vi "Skip Header.vi"(6 "transpose (yes:T)":bool=TRUE, 8 "delimiter (Tab)":string="\t", 9 "number of rows (all:-1)":i32=-1, 10 "number of header lines":i32, 11 "Input File Name":path) -> (0 "Header":string, 1 "header length":i32, 3 "all rows":dbl[][](array[numeric]) format="%_5e", 5 "new file path (Not A Path if cancelled)":path)   [LabVIEW 2018]
uses:
  <vilib>/Utility/file.llb/Read From Spreadsheet File (DBL).vi
panel:
  in  "Numeric":dbl
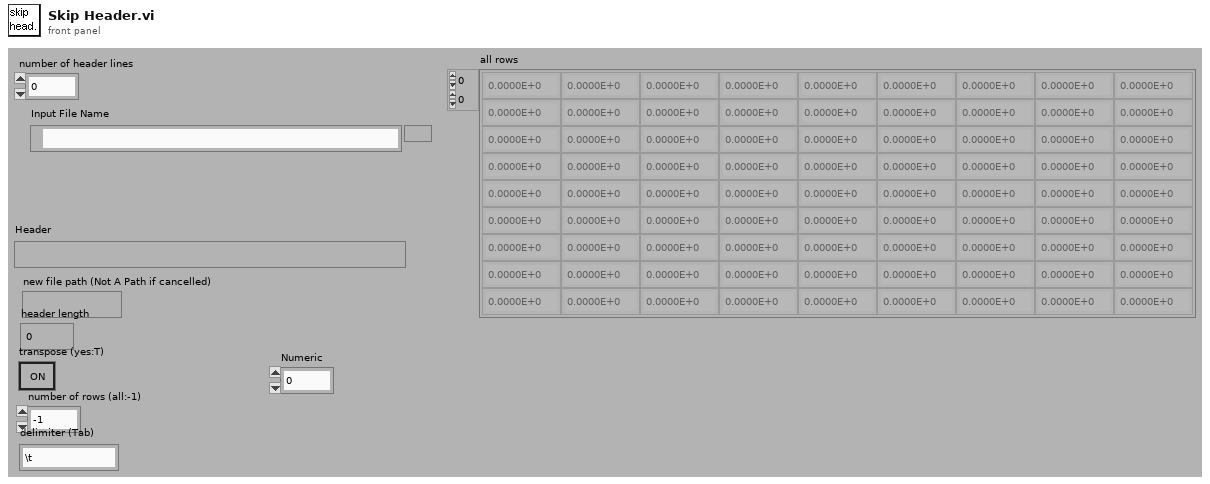
[diagram p1: front panel]
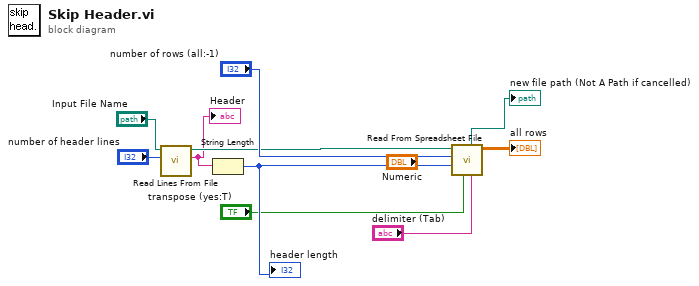
[diagram p0: block diagram]
diagram:
  n1 = call <vilib>:"Read Lines From File.vi"("file path (dialog if empty)"="Input File Name", "number of lines (all:-1)"="number of header lines") -> ("new file path (Not A Path if cancelled)"=w3:path, "line string"=w1:string)  [unwired: 6 out]
  "Header" <- w1
  n2 = String Length(string=w1) -> (length=w6:i32)
  "header length" <- w6
  n3 = call-poly <vilib>:"Read From Spreadsheet File.vi"("delimiter (\\t)"="delimiter (Tab)", "transpose (no:F)"="transpose (yes:T)", "start of read offset (chars.:0)"=w6, "number of rows (all:-1)"="number of rows (all:-1)", "file path (dialog if empty)"=w3) -> ("all rows"=→"all rows":dbl[][], "new file path (Not A Path if cancelled)"=→"new file path (Not A Path if cancelled)":path)  [unwired: 1 in, 4 out]
